vi "Get Interface.vi"(8 "error in (no error)":errorcluster, 11 "index":i32) -> (0 "error out":errorcluster, 2 "lvwpcap_interface_array":string[](array[string]))   [LabVIEW 2025, in "Automotive Ethernet Bus Monitor UI.lvlib" / "lvwpcap.lvlib"]
doc: "This VI outputs the names and descriptions for each ethernet adapter in your system."
uses:
  lvwpcap.lvlib
  lvwpcap.dll
panel:
  # "Select Help»Show Context Help and move the cursor over the VI icon to display help for this VI."
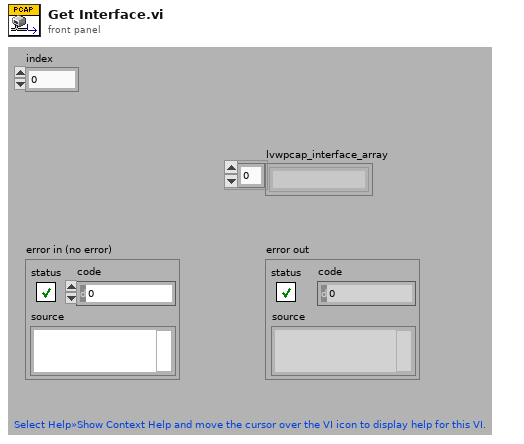
[diagram p1: front panel]
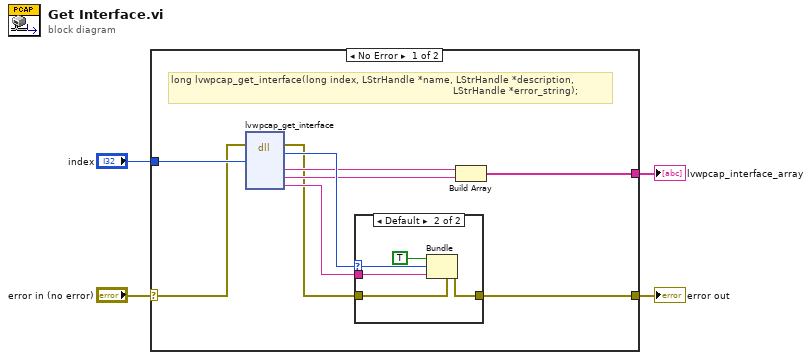
[diagram p0: block diagram]
diagram:
  n1 = case shown="No Error" "error in (no error)" {
    selector: "error in (no error)" -> [w6 w20]
    tunnel: [w13 w20] -> w4
    tunnel: [w8 _] -> w2
    tunnel: "index" -> [w7 _]
    frame No Error {
      # "long lvwpcap_get_interface(long index, LStrHandle *name, LStrHandle *description,\n                                                                                              LStrHandle *error_string);"
      n2 = dll-call lib="lvwpcap.*" fn="lvwpcap_get_interface"(error in=w6, "index"=w7) -> (error out=w5:errorcluster, "return type"=w12:i32, "name"=w10:string, "description"=w9:string, "error_string"=w11:string)  [unwired: 6 in, 1 out]
      n3 = case shown="Default" w12 {
        selector: w12 -> [_ w18]
        tunnel: w11 -> [_ w17]
        tunnel: w5 -> [w14 w19]
        tunnel: [w14 w15] -> w13
        frame 0 {
        }
        frame Default {
          n4 = Bundle(cluster=w19, "status"=TRUE, "code"=w18, "source"=w17) -> (w15:errorcluster)
        }
      }
      n5 = Build Array(w10, w9) -> (w8:string[])
    }
    frame Error {
    }
  }
  "error out" <- w4
  "lvwpcap_interface_array" <- w2
